vi "motors.vi"(10 "stop":bool, 11 "throtel":dbl(knob) scale=0.0..180.0) -> (1 "backword":bool, 2 "left":bool, 3 "RPM":dbl(knob) scale=0.0..180.0, 4 "right":bool, 5 "forward":bool)   [LabVIEW 2013]
uses:
  <vilib>/LabVIEW Interface for Arduino/Type Defs/Board Type.ctl
  <vilib>/LabVIEW Interface for Arduino/Type Defs/Connection Type.ctl
  <vilib>/LabVIEW Interface for Arduino/Type Defs/Pin Mode.ctl
  <vilib>/Utility/inputDevices.llb/closeJoystick.vi
  <vilib>/Utility/inputDevices.llb/joystickAcquire.vi
  <vilib>/LabVIEW Interface for Arduino/LabVIEW Interface for Arduino.lvlib
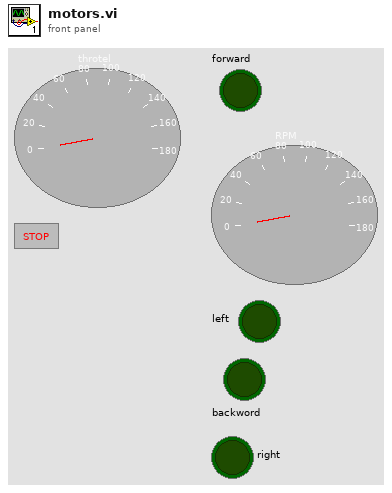
[diagram p1: front panel]
types:
  T1 = typedef "LabVIEW Interface for Arduino.lvlib/Pin Mode.ctl" = enum8{"Input", "Output"}
  T2 = typedef "LabVIEW Interface for Arduino.lvlib/Connection Type.ctl" = enum8{"USB / Serial", "XBEE", "BlueSmirf (Bluetooth)"}
  T3 = typedef "LabVIEW Interface for Arduino.lvlib/Board Type.ctl" = enum16{"Uno", "Dimuelanove w/Atmega 328", "Mega 2560"}
  T4 = typedef "LabVIEW Interface for Arduino.lvlib/Arduino Resource.ctl" = cluster{"VISA resource":refnum<visa-resource-name>, "Board Type":T3, "Connection Type":enum8{"USB / Serial"}, "Bytes Per Packet (15)":u8}
  T5 = cluster{"X axis":i32, "Y axis":i32, "Z axis":i32, "X axis rotation":i32, "Y axis rotation":i32, "Z axis rotation":i32, "U axis":i32, "V axis":i32}
  T6 = cluster{"button 1":bool, "button 2":bool, "button 3":bool, "button 4":bool, "button 5":bool, "button 6":bool, "button 7":bool, "button 8":bool, "button 9":bool, "button 10":bool, "button 11":bool, "button 12":bool, "button 13":bool, "button 14":bool, "button 15":bool, "button 16":bool, "button 17":bool, "button 18":bool, "button 19":bool, "button 20":bool, "button 21":bool, "button 22":bool, "button 23":bool, "button 24":bool, "button 25":bool, "button 26":bool, "button 27":bool, "button 28":bool, "button 29":bool, "button 30":bool, "button 31":bool, "button 32":bool}
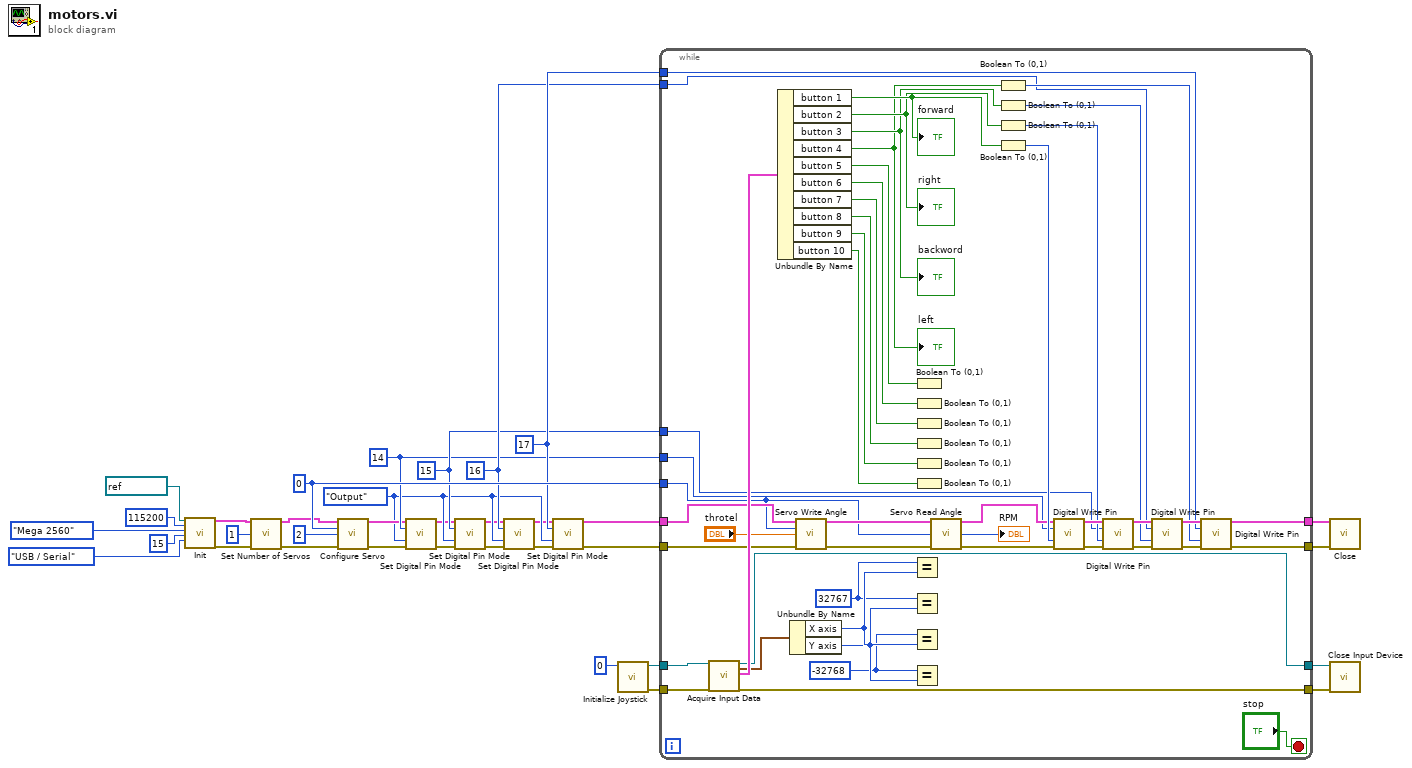
[diagram p0: block diagram]
diagram:
  w31 = u8 17 ("Value (0)")
  w30 = u8 16 ("Value (0)")
  w29 = u8 15 ("Value (0)")
  w28 = u8 14 ("Value (0)")
  w23 = Pin_Mode."Output" ("Pin Mode (Input)")
  w32 = u8 0 ("Servo Number")
  n1 = call <vilib>:"Init.vi"("VISA resource"=refnum<visa-resource-name> "COM9", "Baud Rate (115200)"=u32 115200, "Board Type (Uno)"=Board_Type."Mega 2560", "Bytes Per Packet (15)"=u32 15, "Connection Type (USB/Serial)"=Connection_Type."USB / Serial") -> ("Arduino Resource"=w15:T4, "error out"=w16:errorcluster)  [unwired: 13 in]
  n2 = call <vilib>:"Set Number of Servos.vi"("Arduino Resource"=w15, "Number Of Servos (1)"=u8 1, "error in"=w16) -> ("Arduino Resource"=w11:T4, "error out"=w12:errorcluster)  [unwired: 11 in]
  n3 = call <vilib>:"Configure Servo.vi"("Arduino Resource"=w11, "Servo Number (0)"=w32, "DIO Pin (2)"=u8 2 ("Servo Number"), "error in"=w12) -> ("Arduino Resource"=w26:T4, "error out"=w27:errorcluster)  [unwired: 10 in]
  n4 = call <vilib>:"Set Digital Pin Mode.vi"("Arduino Resource"=w26, "Digital I/O Pin"=w28, "Pin Mode (Input)"=w23, "error in"=w27) -> ("Arduino Resource"=w17:T4, "error out"=w22:errorcluster)  [unwired: 10 in]
  n5 = call <vilib>:"Set Digital Pin Mode.vi"("Arduino Resource"=w17, "Digital I/O Pin"=w29, "Pin Mode (Input)"=w23, "error in"=w22) -> ("Arduino Resource"=w18:T4, "error out"=w21:errorcluster)  [unwired: 10 in]
  n6 = call <vilib>:"Set Digital Pin Mode.vi"("Arduino Resource"=w18, "Digital I/O Pin"=w30, "Pin Mode (Input)"=w23, "error in"=w21) -> ("Arduino Resource"=w19:T4, "error out"=w20:errorcluster)  [unwired: 10 in]
  n7 = call <vilib>:"Set Digital Pin Mode.vi"("Arduino Resource"=w19, "Digital I/O Pin"=w31, "Pin Mode (Input)"=w23, "error in"=w20) -> ("Arduino Resource"=w24:T4, "error out"=w25:errorcluster)  [unwired: 10 in]
  n8 = call <vilib>:"Initialize Joystick.vi"("device index"=0) -> ("error out"=w6:errorcluster, "device ID"=w5:refnum<k1>)  [unwired: 9 in]
  n9 = while {
    tunnel: w5 -> [w79]
    tunnel: w6 -> [w78]
    tunnel: [w36] -> w7
    tunnel: [w35] -> w8
    tunnel: [w71] -> w9
    tunnel: [w70] -> w10
    tunnel: w24 -> [w43]
    tunnel: w25 -> [w42]
    tunnel: w28 -> [w41]
    tunnel: w29 -> [w40]
    tunnel: w30 -> [w39]
    tunnel: w31 -> [w38]
    tunnel: w32 -> [w37]
    stop <- "stop" stop-if-true
    w72 = -32768 ("x")
    w74 = 32767 ("x")
    n10 = call-poly <vilib>:"Acquire Input Data.vi"("device ID"=w79, "error in (no error)"=w78) -> ("device ID"=w71:refnum<k1>, "axis info"=w76:T5, "button info"=w77:T6, "error out"=w70:errorcluster)  [unwired: 13 in, 1 out]
    n11 = Unbundle By Name(w77) -> ("button 1"=w69:bool, "button 2"=w68:bool, "button 3"=w67:bool, "button 4"=w66:bool, "button 5"=w65:bool, "button 6"=w64:bool, "button 7"=w63:bool, "button 8"=w62:bool, "button 9"=w61:bool, "button 10"=w60:bool)
    "forward" <- w69
    "right" <- w68
    "backword" <- w67
    "left" <- w66
    n12 = Unbundle By Name(w76) -> ("X axis"=w75:i32, "Y axis"=w73:i32)
    n13 = call <vilib>:"Servo Write Angle.vi"("Arduino Resource"=w43, "Servo Number"=w37, "Angle (Degrees)"="throtel", "error in"=w42) -> ("Arduino Resource"=w47:T4, "error out"=w46:errorcluster)  [unwired: 10 in]
    n14 = Equal?(x=w74, y=w75) -> ()  [unwired: 1 out]
    n15 = Equal?(x=w74, y=w73) -> ()  [unwired: 1 out]
    n16 = Equal?(x=w72, y=w75) -> ()  [unwired: 1 out]
    n17 = Equal?(x=w72, y=w73) -> ()  [unwired: 1 out]
    n18 = Boolean To (0,1)(Boolean=w65) -> ()  [unwired: 1 out]
    n19 = Boolean To (0,1)(Boolean=w64) -> ()  [unwired: 1 out]
    n20 = Boolean To (0,1)(Boolean=w63) -> ()  [unwired: 1 out]
    n21 = Boolean To (0,1)(Boolean=w62) -> ()  [unwired: 1 out]
    n22 = Boolean To (0,1)(Boolean=w61) -> ()  [unwired: 1 out]
    n23 = Boolean To (0,1)(Boolean=w60) -> ()  [unwired: 1 out]
    n24 = call <vilib>:"Servo Read Angle.vi"("Arduino Resource"=w47, "Servo Number"=w37, "error in"=w46) -> ("Arduino Resource"=w45:T4, "Angle (Degrees)"=→"RPM":u8, "error out"=w44:errorcluster)  [unwired: 10 in]
    n25 = Boolean To (0,1)(Boolean=w66) -> (0, 1=w53:i16)
    n26 = Boolean To (0,1)(Boolean=w67) -> (0, 1=w52:i16)
    n27 = Boolean To (0,1)(Boolean=w68) -> (0, 1=w51:i16)
    n28 = Boolean To (0,1)(Boolean=w69) -> (0, 1=w50:i16)
    n29 = call <vilib>:"Digital Write Pin.vi"("Arduino Resource"=w45, "Digital I/O Pin (0)"=w41, "Value (0)"=w50, "error in"=w44) -> ("Arduino Resource"=w54:T4, "error out"=w57:errorcluster)  [unwired: 10 in]
    n30 = call <vilib>:"Digital Write Pin.vi"("Arduino Resource"=w54, "Digital I/O Pin (0)"=w40, "Value (0)"=w51, "error in"=w57) -> ("Arduino Resource"=w59:T4, "error out"=w56:errorcluster)  [unwired: 10 in]
    n31 = call <vilib>:"Digital Write Pin.vi"("Arduino Resource"=w59, "Digital I/O Pin (0)"=w39, "Value (0)"=w52, "error in"=w56) -> ("Arduino Resource"=w58:T4, "error out"=w55:errorcluster)  [unwired: 10 in]
    n32 = call <vilib>:"Digital Write Pin.vi"("Arduino Resource"=w58, "Digital I/O Pin (0)"=w38, "Value (0)"=w53, "error in"=w55) -> ("Arduino Resource"=w36:T4, "error out"=w35:errorcluster)  [unwired: 10 in]
  }
  n33 = call <vilib>:"Close.vi"("Arduino Resource"=w7, "error in"=w8) -> ()  [unwired: 13 in, 1 out]
  n34 = call-poly <vilib>:"Close Input Device.vi"("error in (no error)"=w10, "device ID"=w9) -> ()  [unwired: 8 in, 1 out]
